vi "VI Tester Menu Selection.vi"(8 "error in":errorcluster, 9 "Config In":variant, 10 "Shortcut Menu Selection":T1, 11 "Active VI Info":T2) -> (0 "error out":errorcluster, 1 "Config Out":variant, 2 "Config Changed":bool)   [LabVIEW 2009]
uses:
  <vilib>/addons/_JKI Toolkits/RCF API/Right Click API.llb/Framework - Active VI Info - Cluster - __RightClickAPI.ctl
  <vilib>/addons/_JKI Toolkits/RCF API/Right Click API.llb/Framework - Selection Type - Enum - __RightClickAPI.ctl
  <vilib>/addons/_JKI Toolkits/RCF API/Right Click API.llb/Framework - Shortcut Menu Selection Events - Cluster - __RightClickAPI.ctl
  <userlib>/_OpenG.lib/array/array.llb/Filter 1D Array (String)__ogtk.vi
  <vilib>/addons/_JKI Toolkits/RCF API/Right Click API.llb/RightClickAPI.lvlib
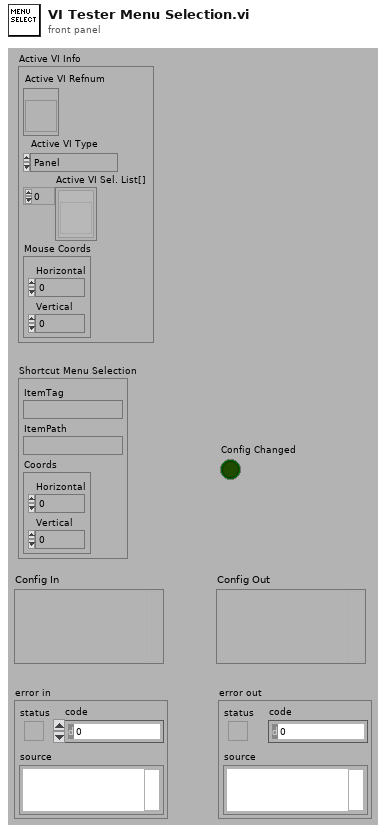
[diagram p1: front panel]
types:
  T1 = typedef "RightClickAPI.lvlib/Framework - Shortcut Menu Selection Events - Cluster - __RightClickAPI.ctl" = cluster{"ItemTag":string, "ItemPath":string, "Coords":cluster{"Horizontal":i32, "Vertical":i32}}
  T2 = typedef "RightClickAPI.lvlib/Framework - Active VI Info - Cluster - __RightClickAPI.ctl" = cluster{"Active VI Refnum":refnum<vi>, "Active VI Type":T3, "Active VI Sel. List[]":refnum<vi>[], "Mouse Coords":cluster{"Horizontal":i32, "Vertical":i32}}
  T3 = typedef "RightClickAPI.lvlib/Framework - Selection Type - Enum - __RightClickAPI.ctl" = enum16{"Panel", "Diagram"}
  T4 = cluster{"Last Test":string, "Recent Tests":string, "Test Template Path (\"\": Use VI Tester Default)":path}
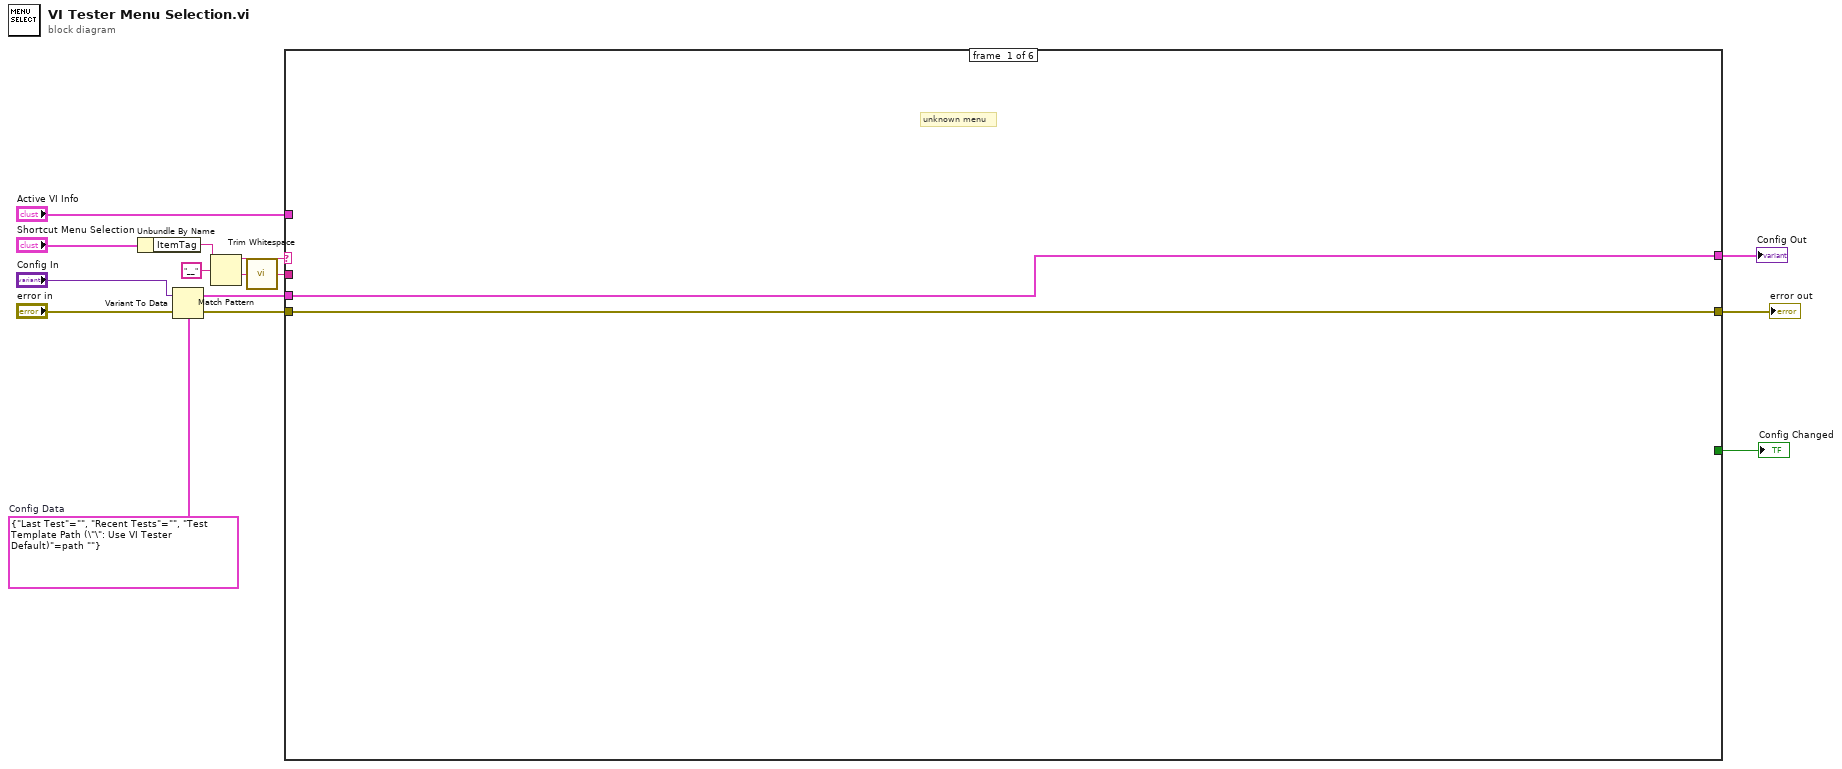
[diagram p0: block diagram]
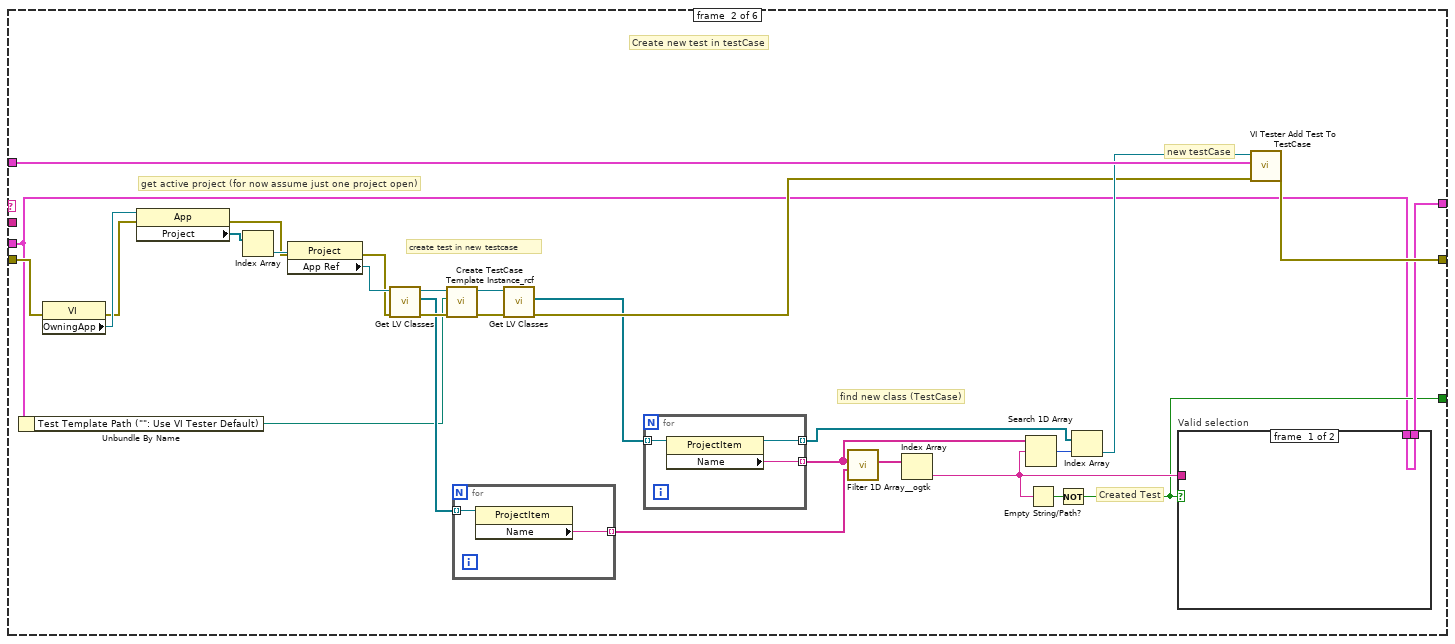
[diagram p2: hidden frame]
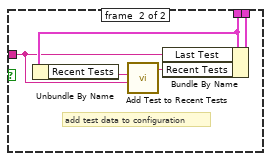
[diagram p3: hidden frame]
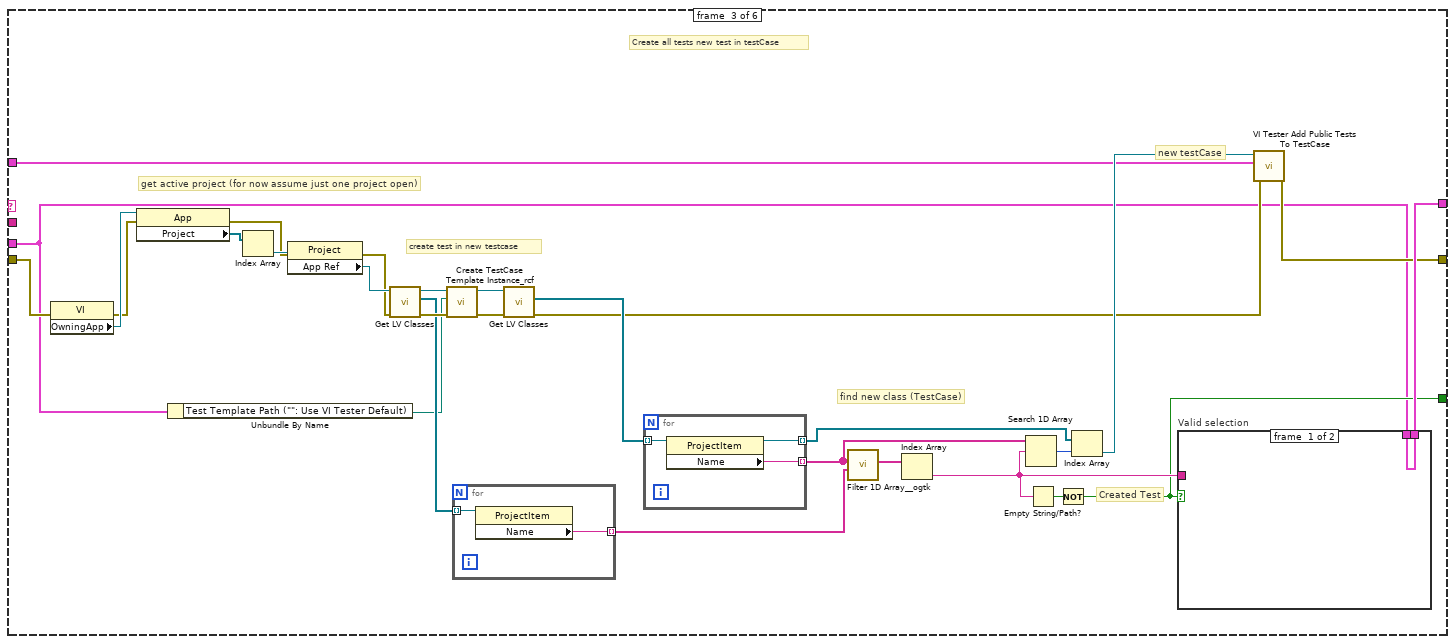
[diagram p4: hidden frame]
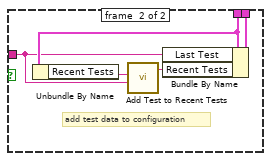
[diagram p5: hidden frame]
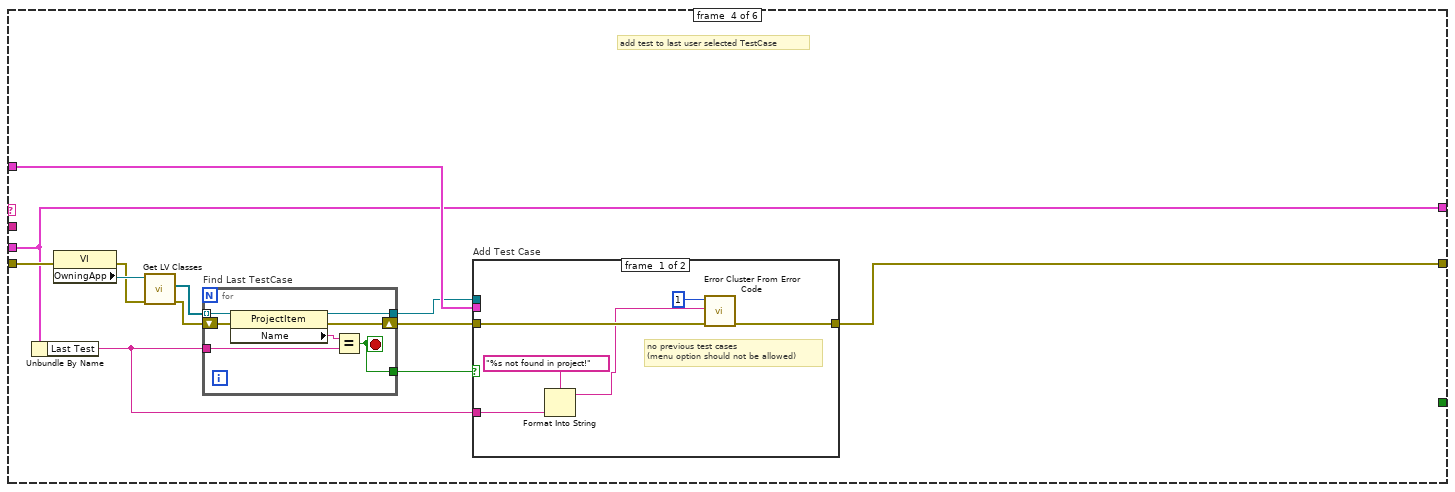
[diagram p6: hidden frame]
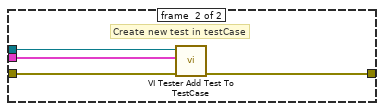
[diagram p7: hidden frame]
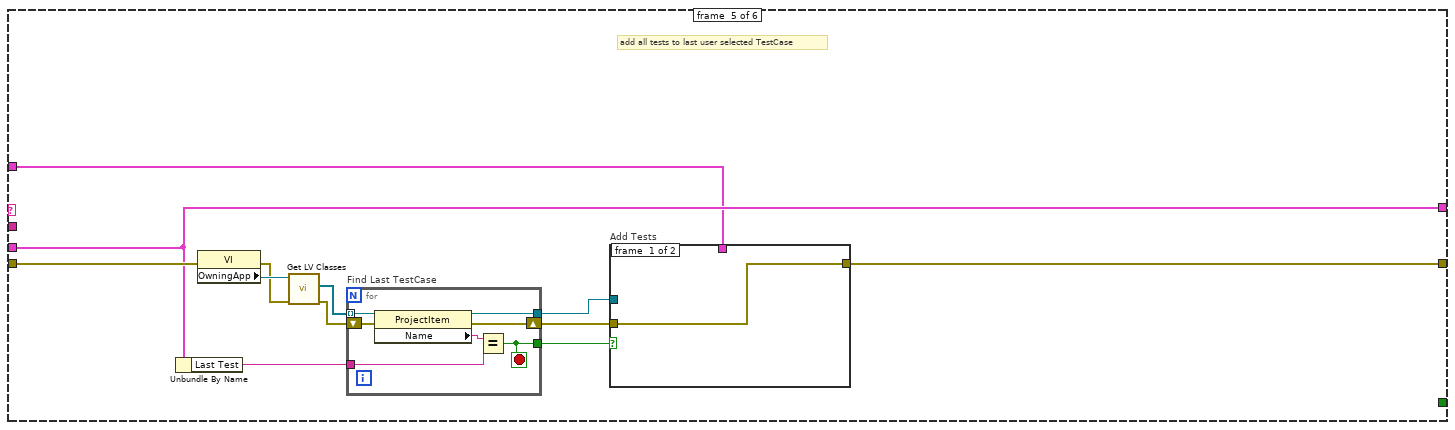
[diagram p8: hidden frame]
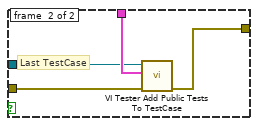
[diagram p9: hidden frame]
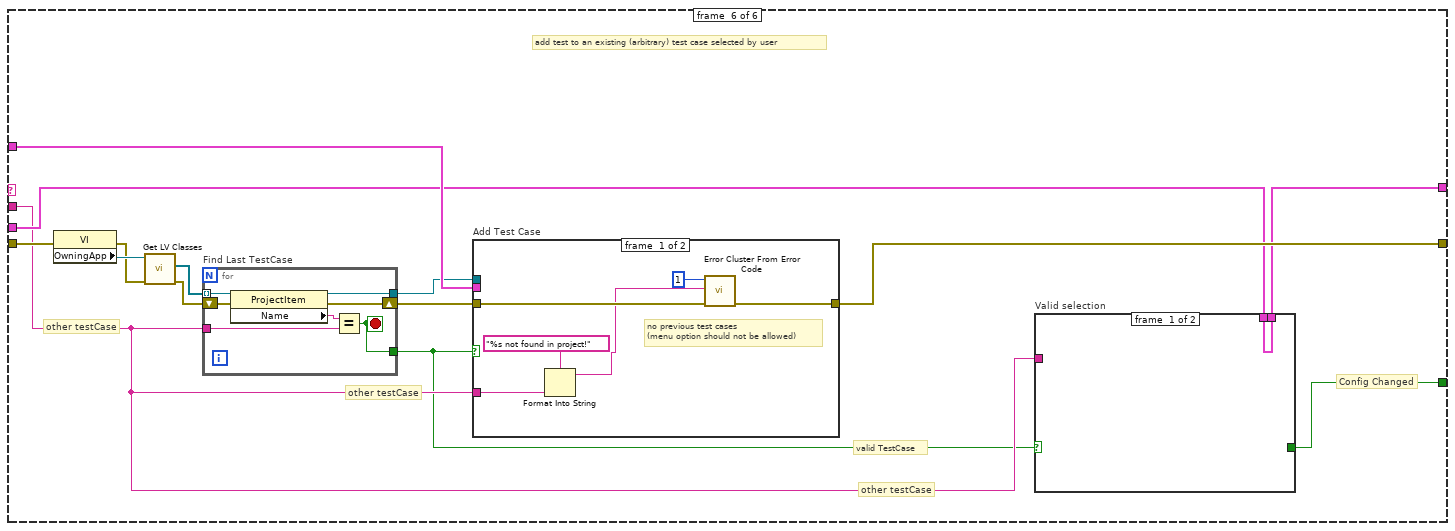
[diagram p10: hidden frame]
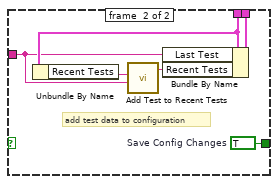
[diagram p11: hidden frame]
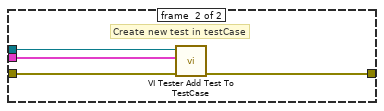
[diagram p12: hidden frame]
diagram:
  w1 = T4 {"Last Test"="", "Recent Tests"="", "Test Template Path (\"\": Use VI Tester Default)"=path ""}  # Config Data
  n1 = Unbundle By Name("Shortcut Menu Selection") -> ("ItemTag"=w5:string)
  n2 = Variant To Data(error in="error in", Variant="Config In", type=w1) -> (error out=w10:errorcluster, data=w9:T4)
  n3 = Match Pattern(string=w5, regular expression="__") -> (before substring=w4:string, after substring=w3:string)  [unwired: 1 in, 2 out]
  n4 = call <vilib>:"Trim Whitespace.vi"("string"=w3) -> ("trimmed string"=w2:string)  [unwired: 1 in]
  n5 = case shown="\"append in other test\"" w4 {
    tunnel: [w17 w45 w60 w107 w138 w162] -> w14
    tunnel: w10 -> [w17 w35 w78 w105 w136 w160]
    tunnel: "Active VI Info" -> [_ w46 w62 w109 w130 w164]
    tunnel: w9 -> [w16 w19 w59 w98 w131 w155]
    tunnel: [w16 w26 w70 w98 w131 w154] -> w8
    tunnel: [_ w23 w67 _ _ w151] -> w7
    tunnel: w2 -> [_ _ _ _ _ w153]
    frame #0 {
      # "unknown menu"
    }
    frame #1 {
      # "Created Test"
      # "Create new test in testCase"
      # "get active project (for now assume just one project open)"
      # "find new class (TestCase)"
      # "create test in new testcase"
      # "new testCase"
      n6 = Unbundle By Name(w19) -> ("Test Template Path (\"\": Use VI Tester Default)"=w18:path)
      n7 = property class="VI"(error in=w35) -> (error out=w21:errorcluster, "OwningApp"=w28:refnum<vi>)  [unwired: 1 in, 1 out]
      n8 = property class="App"(reference=w28, error in=w21) -> (error out=w22:errorcluster, "Project"=w30:refnum<vi>[])  [unwired: 1 out]
      n9 = Index Array(array=w30) -> (element=w29:refnum<vi>)  [unwired: 1 in]
      n10 = property class="Project"(reference=w29, error in=w22) -> (error out=w20:errorcluster, "App Ref"=w27:refnum<vi>)  [unwired: 1 out]
      n11 = call "Get LV Classes.vi"("error in (no error)"=w20, "App reference"=w27) -> ("error out"=w37:errorcluster, "LabVIEW Classes"=w33:refnum<vi>[], "dup App reference"=w31:refnum<vi>)  [unwired: 7 in]
      n12 = call "Create TestCase Template Instance_rcf.vi"("error in"=w37, "Template Class Path"=w18, "Application Ref (This Application)"=w31) -> ("error out"=w36:errorcluster, "Application Ref"=w44:refnum<vi>)  [unwired: 7 in]
      n13 = for {
        tunnel: w33 -> [w57] mode=indexing
        tunnel: [w56] -> w43 mode=indexing
        n14 = property class="ProjectItem"(reference=w57) -> ("Name"=w56:string)  [unwired: 1 in, 2 out]
      }
      n15 = call "Get LV Classes.vi"("error in (no error)"=w36, "App reference"=w44) -> ("error out"=w34:errorcluster, "LabVIEW Classes"=w32:refnum<vi>[])  [unwired: 7 in, 1 out]
      n16 = for {
        tunnel: w32 -> [w55] mode=indexing
        tunnel: [w54] -> w41 mode=indexing
        tunnel: [w53] -> w39 mode=indexing
        n17 = property class="ProjectItem"(reference=w55) -> (reference out=w53:refnum<vi>, "Name"=w54:string)  [unwired: 1 in, 1 out]
      }
      n18 = call-poly <userlib>:"Filter 1D Array__ogtk.vi"("items to filter"=w43, "array"=w41) -> ("filtered array"=w42:string[])  [unwired: 4 in, 1 out]
      n19 = Index Array(array=w42) -> (element=w25:string)  [unwired: 1 in]
      n20 = Search 1D Array(1D array=w41, element=w25) -> (index of element=w40:i32)  [unwired: 1 in]
      n21 = Empty String/Path?(string/path=w25) -> (empty?=w24:bool)
      n22 = Not(x=w24) -> (.not. x?=w23:bool)
      n23 = Index Array(array=w39, index=w40) -> (element=w38:refnum<vi>)
      n24 = case "Valid selection" shown="True" w23 {
        tunnel: w19 -> [w47 w51]
        tunnel: [w47 w52] -> w26
        tunnel: w25 -> [_ w49]
        frame #0 {
        }
        frame #1 {
          # "add test data to configuration"
          n25 = Unbundle By Name(w51) -> ("Recent Tests"=w50:string)
          n26 = call "Add Test to Recent Tests.vi"("New Test"=w49, "Recent Tests"=w50) -> ("Recent Tests"=w48:string)  [unwired: 9 in]
          n27 = Bundle By Name(cluster=w51, "Last Test"=w49, "Recent Tests"=w48) -> (w52:T4)
        }
      }
      n28 = call "VI Tester Add Test To TestCase.vi"("error in"=w34, "Active VI Info"=w46, "TestCase Refnum"=w38) -> ("error out"=w45:errorcluster)  [unwired: 8 in]
    }
    frame #2 {
      # "Created Test"
      # "Create all tests new test in testCase"
      # "get active project (for now assume just one project open)"
      # "find new class (TestCase)"
      # "create test in new testcase"
      # "new testCase"
      n29 = property class="VI"(error in=w78) -> (error out=w65:errorcluster, "OwningApp"=w72:refnum<vi>)  [unwired: 1 in, 1 out]
      n30 = property class="App"(reference=w72, error in=w65) -> (error out=w66:errorcluster, "Project"=w74:refnum<vi>[])  [unwired: 1 out]
      n31 = Unbundle By Name(w59) -> ("Test Template Path (\"\": Use VI Tester Default)"=w58:path)
      n32 = Index Array(array=w74) -> (element=w73:refnum<vi>)  [unwired: 1 in]
      n33 = property class="Project"(reference=w73, error in=w66) -> (error out=w64:errorcluster, "App Ref"=w71:refnum<vi>)  [unwired: 1 out]
      n34 = call "Get LV Classes.vi"("error in (no error)"=w64, "App reference"=w71) -> ("error out"=w80:errorcluster, "LabVIEW Classes"=w77:refnum<vi>[], "dup App reference"=w75:refnum<vi>)  [unwired: 7 in]
      n35 = call "Create TestCase Template Instance_rcf.vi"("error in"=w80, "Template Class Path"=w58, "Application Ref (This Application)"=w75) -> ("error out"=w79:errorcluster, "Application Ref"=w86:refnum<vi>)  [unwired: 7 in]
      n36 = for {
        tunnel: w77 -> [w97] mode=indexing
        tunnel: [w96] -> w85 mode=indexing
        n37 = property class="ProjectItem"(reference=w97) -> ("Name"=w96:string)  [unwired: 1 in, 2 out]
      }
      n38 = call "Get LV Classes.vi"("error in (no error)"=w79, "App reference"=w86) -> ("error out"=w61:errorcluster, "LabVIEW Classes"=w76:refnum<vi>[])  [unwired: 7 in, 1 out]
      n39 = for {
        tunnel: w76 -> [w95] mode=indexing
        tunnel: [w94] -> w83 mode=indexing
        tunnel: [w93] -> w81 mode=indexing
        n40 = property class="ProjectItem"(reference=w95) -> (reference out=w93:refnum<vi>, "Name"=w94:string)  [unwired: 1 in, 1 out]
      }
      n41 = call-poly <userlib>:"Filter 1D Array__ogtk.vi"("items to filter"=w85, "array"=w83) -> ("filtered array"=w84:string[])  [unwired: 4 in, 1 out]
      n42 = Index Array(array=w84) -> (element=w69:string)  [unwired: 1 in]
      n43 = Search 1D Array(1D array=w83, element=w69) -> (index of element=w82:i32)  [unwired: 1 in]
      n44 = Empty String/Path?(string/path=w69) -> (empty?=w68:bool)
      n45 = Not(x=w68) -> (.not. x?=w67:bool)
      n46 = Index Array(array=w81, index=w82) -> (element=w63:refnum<vi>)
      n47 = case "Valid selection" shown="True" w67 {
        tunnel: w59 -> [w87 w91]
        tunnel: [w87 w92] -> w70
        tunnel: w69 -> [_ w89]
        frame #0 {
        }
        frame #1 {
          # "add test data to configuration"
          n48 = Unbundle By Name(w91) -> ("Recent Tests"=w90:string)
          n49 = call "Add Test to Recent Tests.vi"("New Test"=w89, "Recent Tests"=w90) -> ("Recent Tests"=w88:string)  [unwired: 9 in]
          n50 = Bundle By Name(cluster=w91, "Last Test"=w89, "Recent Tests"=w88) -> (w92:T4)
        }
      }
      n51 = call "VI Tester Add Public Tests To TestCase.vi"("error in"=w61, "Active VI Info"=w62, "TestCase Refnum"=w63) -> ("error out"=w60:errorcluster)  [unwired: 8 in]
    }
    frame #3 {
      # "add test to last user selected TestCase"
      n52 = Unbundle By Name(w98) -> ("Last Test"=w100:string)
      n53 = property class="VI"(error in=w105) -> (error out=w104:errorcluster, "OwningApp"=w106:refnum<vi>)  [unwired: 1 in, 1 out]
      n54 = call "Get LV Classes.vi"("error in (no error)"=w104, "App reference"=w106) -> ("error out"=w103:errorcluster, "LabVIEW Classes"=w99:refnum<vi>[])  [unwired: 7 in, 1 out]
      n55 = for "Find Last TestCase" {
        tunnel: w99 -> [w126] mode=indexing
        tunnel: w100 -> [w124]
        tunnel: [w123] -> w108
        shift-right: [w121] -> w102
        shift-left: w103 -> [w122]
        tunnel: [w120] -> w101
        stop <- w120 stop-if-true
        n56 = property class="ProjectItem"(reference=w126, error in=w122) -> (reference out=w123:refnum<vi>, error out=w121:errorcluster, "Name"=w125:string)
        n57 = Equal?(x=w125, y=w124) -> (x = y?=w120:bool)
      }
      n58 = case "Add Test Case" shown="True" w101 {
        tunnel: w109 -> [_ w119]
        tunnel: w108 -> [_ w118]
        tunnel: [w114 w117] -> w107
        tunnel: w102 -> [w115 w116]
        tunnel: w100 -> [w112 _]
        frame #0 {
          # "no previous test cases\n(menu option should not be allowed)"
          n59 = Format Into String(format string="%s not found in project!", w112) -> (resulting string=w110:string)  [unwired: 2 in, 1 out]
          n60 = call <vilib>:"Error Cluster From Error Code.vi"("error in (no error)"=w115, "error message (\"\")"=w110, "error code (0)"=1) -> ("error out"=w114:errorcluster)  [unwired: 6 in]
        }
        frame #1 {
          # "Create new test in testCase"
          n61 = call "VI Tester Add Test To TestCase.vi"("error in"=w116, "Active VI Info"=w119, "TestCase Refnum"=w118) -> ("error out"=w117:errorcluster)  [unwired: 8 in]
        }
      }
    }
    frame #4 {
      # "add all tests to last user selected TestCase"
      n62 = Unbundle By Name(w131) -> ("Last Test"=w133:string)
      n63 = property class="VI"(error in=w136) -> (error out=w135:errorcluster, "OwningApp"=w137:refnum<vi>)  [unwired: 1 in, 1 out]
      n64 = call "Get LV Classes.vi"("error in (no error)"=w135, "App reference"=w137) -> ("error out"=w134:errorcluster, "LabVIEW Classes"=w132:refnum<vi>[])  [unwired: 7 in, 1 out]
      n65 = for "Find Last TestCase" {
        tunnel: w132 -> [w150] mode=indexing
        tunnel: w133 -> [w148]
        tunnel: [w147] -> w129
        shift-right: [w145] -> w128
        shift-left: w134 -> [w146]
        tunnel: [w144] -> w127
        stop <- w144 stop-if-true
        n66 = property class="ProjectItem"(reference=w150, error in=w146) -> (reference out=w147:refnum<vi>, error out=w145:errorcluster, "Name"=w149:string)
        n67 = Equal?(x=w149, y=w148) -> (x = y?=w144:bool)
      }
      n68 = case "Add Tests" shown="True" w127 {
        tunnel: [w139 w143] -> w138
        tunnel: w130 -> [_ w142]
        tunnel: w129 -> [_ w141]
        tunnel: w128 -> [w139 w140]
        frame #0 {
        }
        frame #1 {
          # "Last TestCase"
          n69 = call "VI Tester Add Public Tests To TestCase.vi"("error in"=w140, "Active VI Info"=w142, "TestCase Refnum"=w141) -> ("error out"=w143:errorcluster)  [unwired: 8 in]
        }
      }
    }
    frame #5 {
      # "add test to an existing (arbitrary) test case selected by user"
      # "Config Changed"
      # "valid TestCase"
      # "other testCase"
      # "other testCase"
      # "other testCase"
      n70 = property class="VI"(error in=w160) -> (error out=w159:errorcluster, "OwningApp"=w161:refnum<vi>)  [unwired: 1 in, 1 out]
      n71 = call "Get LV Classes.vi"("error in (no error)"=w159, "App reference"=w161) -> ("error out"=w158:errorcluster, "LabVIEW Classes"=w156:refnum<vi>[])  [unwired: 7 in, 1 out]
      n72 = for "Find Last TestCase" {
        tunnel: w156 -> [w188] mode=indexing
        tunnel: w153 -> [w186]
        tunnel: [w185] -> w163
        shift-right: [w183] -> w157
        shift-left: w158 -> [w184]
        tunnel: [w182] -> w152
        stop <- w182 stop-if-true
        n73 = property class="ProjectItem"(reference=w188, error in=w184) -> (reference out=w185:refnum<vi>, error out=w183:errorcluster, "Name"=w187:string)
        n74 = Equal?(x=w187, y=w186) -> (x = y?=w182:bool)
      }
      n75 = case "Add Test Case" shown="True" w152 {
        tunnel: w164 -> [_ w181]
        tunnel: w163 -> [_ w180]
        tunnel: [w176 w179] -> w162
        tunnel: w157 -> [w177 w178]
        tunnel: w153 -> [w174 _]
        frame #0 {
          # "no previous test cases\n(menu option should not be allowed)"
          n76 = Format Into String(format string="%s not found in project!", w174) -> (resulting string=w172:string)  [unwired: 2 in, 1 out]
          n77 = call <vilib>:"Error Cluster From Error Code.vi"("error in (no error)"=w177, "error message (\"\")"=w172, "error code (0)"=1) -> ("error out"=w176:errorcluster)  [unwired: 6 in]
        }
        frame #1 {
          # "Create new test in testCase"
          n78 = call "VI Tester Add Test To TestCase.vi"("error in"=w178, "Active VI Info"=w181, "TestCase Refnum"=w180) -> ("error out"=w179:errorcluster)  [unwired: 8 in]
        }
      }
      n79 = case "Valid selection" shown="True" w152 {
        tunnel: w155 -> [w165 w170]
        tunnel: [w165 w171] -> w154
        tunnel: w153 -> [_ w168]
        tunnel: [_ w166] -> w151
        frame #0 {
        }
        frame #1 {
          w166 = TRUE  # Save Config Changes
          # "add test data to configuration"
          n80 = Unbundle By Name(w170) -> ("Recent Tests"=w169:string)
          n81 = call "Add Test to Recent Tests.vi"("New Test"=w168, "Recent Tests"=w169) -> ("Recent Tests"=w167:string)  [unwired: 9 in]
          n82 = Bundle By Name(cluster=w170, "Last Test"=w168, "Recent Tests"=w167) -> (w171:T4)
        }
      }
    }
  }
  "error out" <- w14
  "Config Out" <- w8
  "Config Changed" <- w7
